vi "Check GPS Initialized.vi"(3 "error in (no error)":errorcluster, 5 "Completed NMEA Sentences":string[](array[string])) -> (0 "error out":errorcluster, 1 "Complete NMEA Sentences (Copy)":string[](array[string]), 2 "Satellites Aquired":bool)   [LabVIEW 2009]
uses:
  <vilib>/robotics/Protocols/NMEA/Advanced/Instrument Specific Poly VIs/GPS/Parse GGA Sentence.vi
  <vilib>/robotics/Protocols/NMEA/NMEA API.lvlib
panel:
  out "input array size":i32
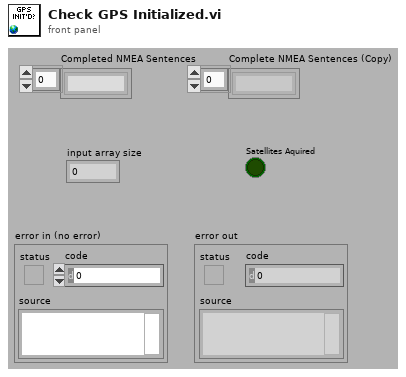
[diagram p1: front panel]
types:
  T1 = typedef "NMEA API.lvlib/GGA Data.ctl" = cluster{"time of fix":cluster{"included?":bool, "time (UTC)":timestamp}, "latitude":cluster{"included?":bool, "latitude (deg)":dbl}, "longitude":cluster{"included?":bool, "longitude (deg)":dbl}, "fix quality":cluster{"included?":bool, "quality":u16}, "number of satellites in view":cluster{"included?":bool, "number of satellites":i8}, "horizontal dilution of precision":cluster{"included?":bool, "horizontal DOP":dbl}, "altitude above mean sea level":cluster{"included?":bool, "altitude (m)":dbl}, "height of geoid above WGS84":cluster{"included?":bool, "height of geoid (m)":dbl}, "time since last DGPS update":cluster{"included?":bool, "time (s)":dbl}, "DGPS station ID number":cluster{"included?":bool, "station ID number":dbl}}
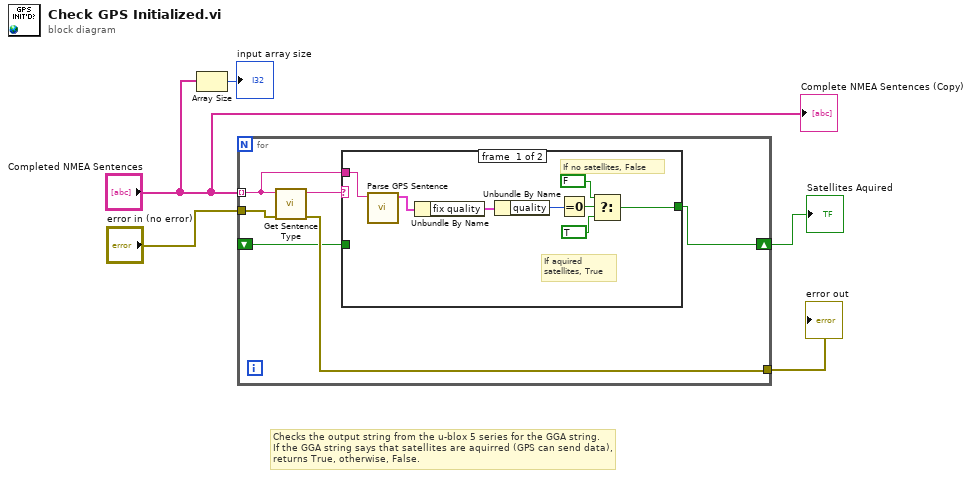
[diagram p0: block diagram]
diagram:
  # "Checks the output string from the u-blox 5 series for the GGA string.\nIf the GGA string says that satellites are aquirred (GPS can send data),\nreturns True, otherwise, False."
  n1 = Array Size(array="Completed NMEA Sentences") -> (size(s)=→"input array size":i32)
  n2 = for {
    tunnel: "Completed NMEA Sentences" -> [w9] mode=indexing
    tunnel: "error in (no error)" -> [w11]
    tunnel: [w8] -> w2
    shift-right: [w7] -> w1
    shift-left: _ -> [w6]
    n3 = call <vilib>:"Get Sentence Type.vi"("error in (no error)"=w11, "sentence"=w9) -> ("error out"=w8:errorcluster, "sentence type"=w10:string)  [unwired: 7 in, 1 out]
    n4 = case shown="\"GPGGA\"" w10 {
      tunnel: w9 -> [w17 _]
      tunnel: [w12 w20] -> w7
      tunnel: w6 -> [_ w20]
      frame #0 {
        # "If no satellites, False"
        # "If aquired \nsatellites, True"
        n5 = call-poly <vilib>:"Parse GPS Sentence.vi"("GGA sentence"=w17) -> ("GGA data"=w19:T1)  [unwired: 9 in, 1 out]
        n6 = Unbundle By Name(w19) -> ("fix quality"=w18:cluster{"included?":bool, "quality":u16})
        n7 = Unbundle By Name(w18) -> ("quality"=w13:u16)
        n8 = Equal To 0?(x=w13) -> (x = 0?=w16:bool)
        n9 = Select(t=FALSE, s=w16, f=TRUE) -> (s? t:f=w12:bool)
      }
      frame #1 {
      }
    }
  }
  "Satellites Aquired" <- w1
  "error out" <- w2
  "Complete NMEA Sentences (Copy)" <- "Completed NMEA Sentences"
